vi "Apply Configuration.vi"(8 "error in (no error)":errorcluster, 11 "Camera Base in":refnum<class "Camera Base.lvclass">) -> (0 "error out":errorcluster, 3 "Camera Base out":refnum<class "Camera Base.lvclass">)   [LabVIEW 2023, in "Camera Base.lvclass"]
uses:
  Camera Base.lvclass
  Camera Base.lvclass/Camera Base.ctl
  Interfaces/IConfigure/IConfigure.lvclass
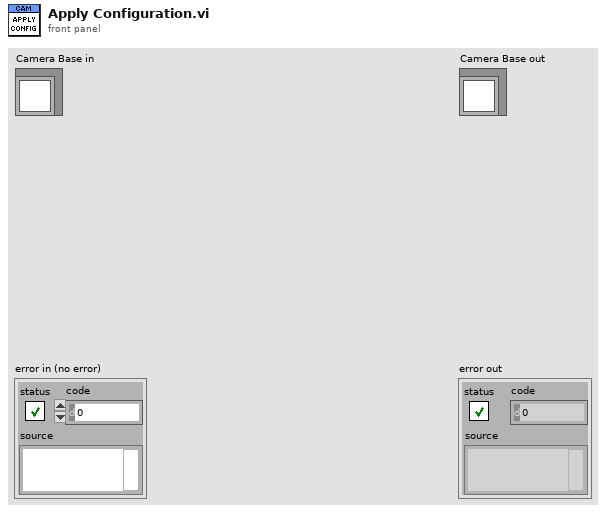
[diagram p1: front panel]
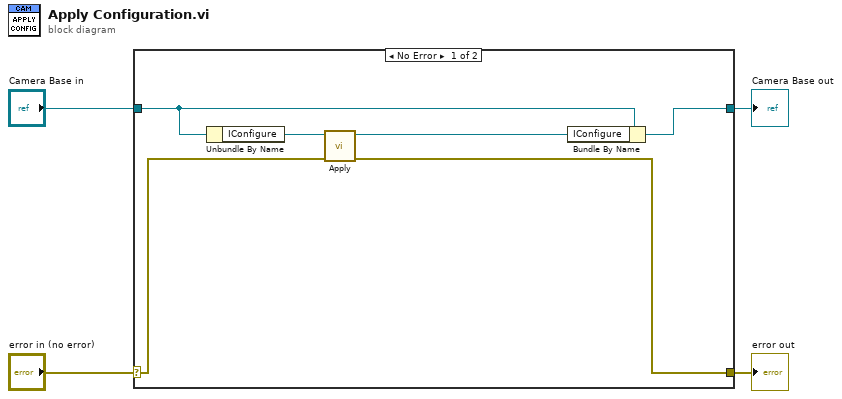
[diagram p0: block diagram]
diagram:
  n1 = case shown="No Error" "error in (no error)" {
    selector: "error in (no error)" -> [w9 w12]
    tunnel: [w8 w12] -> w3
    tunnel: [w7 w11] -> w1
    tunnel: "Camera Base in" -> [w6 w11]
    frame No Error {
      n2 = Unbundle By Name(w6) -> ("IConfigure"=w10:refnum<class "IConfigure.lvclass">)
      n3 = call-dynamic "Apply.vi"("Error In"=w9, "IConfigure in"=w10) -> ("Error Out"=w8:errorcluster, "IConfigure out"=w5:refnum<class "IConfigure.lvclass">)  [unwired: 8 in]
      n4 = Bundle By Name(cluster=w6, "IConfigure"=w5) -> (w7:refnum<class "Camera Base.lvclass">)
    }
    frame Error {
    }
  }
  "error out" <- w3
  "Camera Base out" <- w1
